vi "Open_Refs.vi"(10 "Refs_Destination_Cabine":refnum<vi>[](array[refnum]), 11 "Ref_Appel_Couloir":refnum<vi>[](array[refnum])) -> (3 "Donnees_Globale_Out":T1)   [LabVIEW 2019]
uses:
  Asc_State_Inputs.ctl
  Etat_Asc.ctl
  <vilib>/FPGAPlugInAG/myRIO-1900/niLvFpga_Open_myRIO-1900.vi
  <vilib>/rvi/interface/common/dynamic/niFpgaDynamicAddResources.vi
  <vilib>/Utility/error.llb/Error Cluster From Error Code.vi
  <vilib>/rvi/errors/niLvFpgaAdjustHostInterfaceError.vi
  <vilib>/rvi/interface/nirviOpenFPGA/nirviOpenFPGA.xnode
  FPGA Bitfiles/ascenceur_FPGATarget_FPGAMain_7v9Jr2n8zuw.lvbitx
  L298N/FPGA_Main.vi
  <vilib>/rvi/interface/nirviReadWriteControl/nirviReadWriteControl.xnode
  <vilib>/myRIO/Common/Instrument Driver Framework/myRIO v1.0/DIO/typedefs/DIO Channels Enum.ctl
  <vilib>/myRIO/Common/Instrument Driver Framework/myRIO v1.0/DIO/typedefs/DIO Channels List.ctl
  <vilib>/myRIO/Common/Instrument Driver Framework/Utilities/typedefs/Generic FPGA Reference.ctl
  <vilib>/myRIO/Common/Instrument Driver Framework/Utilities/typedefs/myRIO v1.0 Reference.ctl
  <vilib>/myRIO/Common/Instrument Driver Framework/Utilities/typedefs/Hardware Version Enum.ctl
  <vilib>/myRIO/Common/Instrument Driver Framework/Utilities/typedefs/myRIO Generic Hardware Reference.ctl
  <vilib>/myRIO/Instrument Drivers/Onboard IO/DIO/typedefs/DIO Reference.ctl
  <vilib>/myRIO/Instrument Drivers/Onboard IO/DIO/DIO.lvlib
  <vilib>/userDefined/High Color/nirio_resource_hc.ctl
  <vilib>/myRIO/Common/Instrument Driver Framework/myRIO v1.0/DIO/vis/myRIO v1.1 Open DIO.vi
  <vilib>/myRIO/Instrument Drivers/Onboard IO/DIO/vis/myRIO DIO Open.xnode
  L298N_Driver/L298N_Ref_Type.ctl
  NiFpgaLv.dll
  <vilib>/rvi/interface/Simulation/niFpgaSimulationCallBeginRW.vi
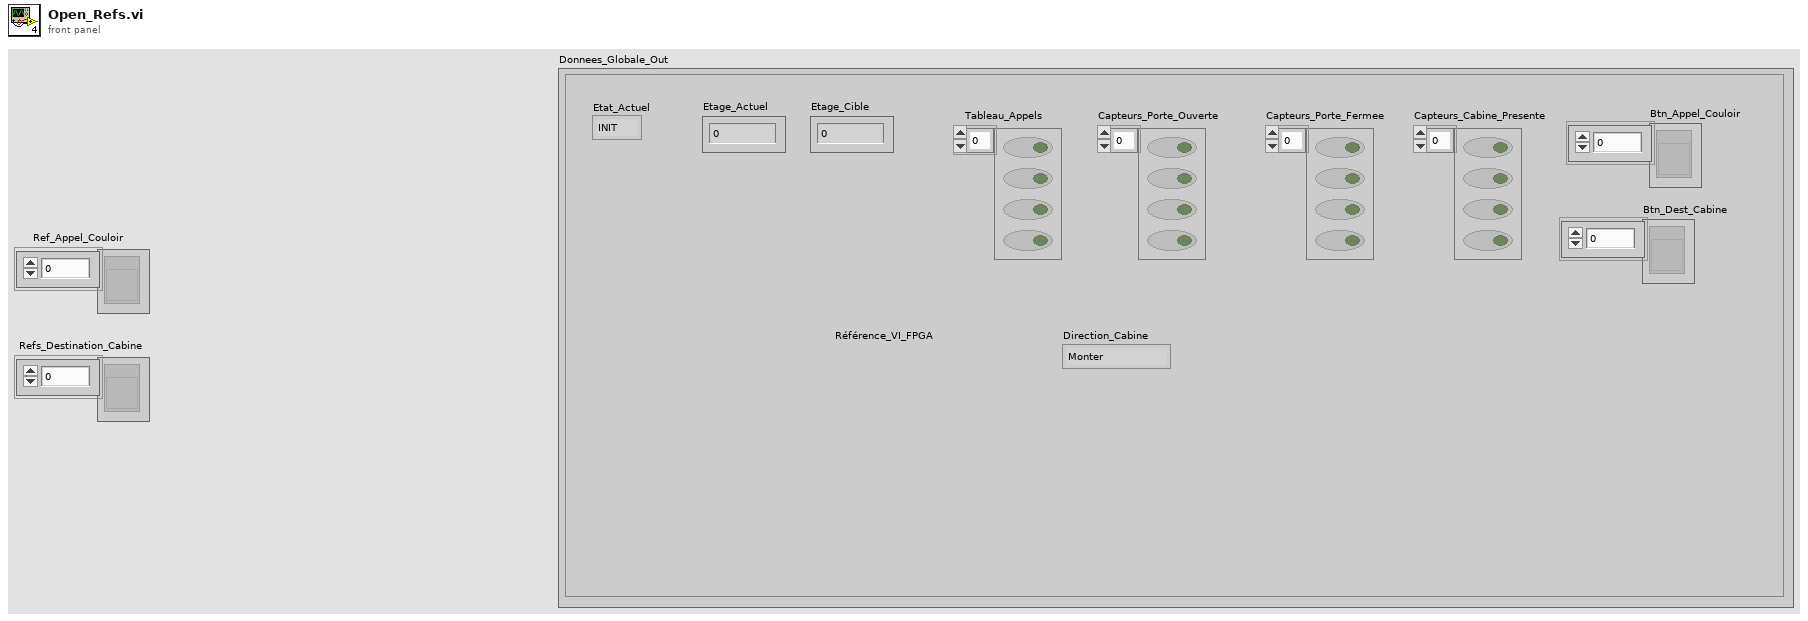
[diagram p1: front panel]
types:
  T1 = typedef "Asc_State_Inputs.ctl" = cluster{"Etage_Actuel":i32, "Etat_Actuel":T2, "Etage_Cible":i32, "Tableau_Appels":bool[], "Capteurs_Porte_Ouverte":bool[], "Capteurs_Porte_Fermee":bool[], "Capteurs_Cabine_Presente":bool[], "Btn_Appel_Couloir":refnum<vi>[], "Btn_Dest_Cabine":refnum<vi>[], "Référence_VI_FPGA":refnum<k20>, "Direction_Cabine":enum16{"Monter", "Descendre", "Arreter"}}
  T2 = typedef "Etat_Asc.ctl" = enum16{"INIT", "REPOS", "DEPLACEMENT", "OUVERTURE_PORTE", "ATTENTE_TEMPO", "FERMETURE_PORTE", "ARRET_URGENCE"}
  T3 = typedef "L298N_Ref_Type.ctl" = cluster{"DIO_Ref_Montee":T4, "DIO_Ref_Descente":T4}
  T4 = typedef "DIO.lvlib/DIO Reference.ctl" = cluster{"myRIO Reference":T5, "DIO Channels List":T9}
  T5 = typedef "myRIO Generic Hardware Reference.ctl" = cluster{"myRIO Model":T6, "myRIO Hardware Reference":T7}
  T6 = typedef "Hardware Version Enum.ctl" = enum16{"Unknown", "myRIO-1900", "myRIO-1950", "roboRIO", "NI ELVIS RIO CM", "ELVIS III"}
  T7 = typedef "myRIO v1.0 Reference.ctl" = cluster{"Generic FPGA Reference":T8, "Allow multiple opens":bool}
  T8 = typedef "Generic FPGA Reference.ctl" = refnum<k20>
  T9 = typedef "DIO Channels List.ctl" = T10[]
  T10 = typedef "DIO Channels Enum.ctl" = enum16{"Not Connected", "C/DIO0", "C/DIO1", "C/DIO2", "C/DIO3", "C/DIO4", "C/DIO5", "C/DIO6", "C/DIO7", "A/DIO0", "A/DIO1", "A/DIO2", "A/DIO3", "A/DIO4", "A/DIO5", "A/DIO6", "A/DIO7", "A/DIO8", "A/DIO9", "A/DIO10", "A/DIO11", "A/DIO12", "A/DIO13", "A/DIO14", "A/DIO15", "A/DIO16", "A/DIO17", "A/DIO18", "A/DIO19", "B/DIO0", "B/DIO1", "B/DIO2", "B/DIO3", "B/DIO4", "B/DIO5", "B/DIO6", "B/DIO7", "B/DIO8", "B/DIO9", "B/DIO10", "B/DIO11", "B/DIO12", "B/DIO13", "B/DIO14", "B/DIO15", "B/DIO16", "B/DIO17", "B/DIO18", "B/DIO19", "LED0", "LED1", "LED2", "LED3", "Button0", "DIO/DIO0", "DIO/DIO1", "DIO/DIO2", "DIO/DIO3", "DIO/DIO4", "DIO/DIO5", "DIO/DIO6", "DIO/DIO7", "DIO/DIO8", "DIO/DIO9", "SPI/CS0", "SPI/CS1", "SPI/CS2", "SPI/CS3", "LED RADIO (Green)", "LED RADIO (Red)", "LED COMM (Green)", "LED COMM (Red)", "LED MODE (Green)", "LED MODE (Red)"}
  T11 = typedef "nirio_resource_hc.ctl" = tag
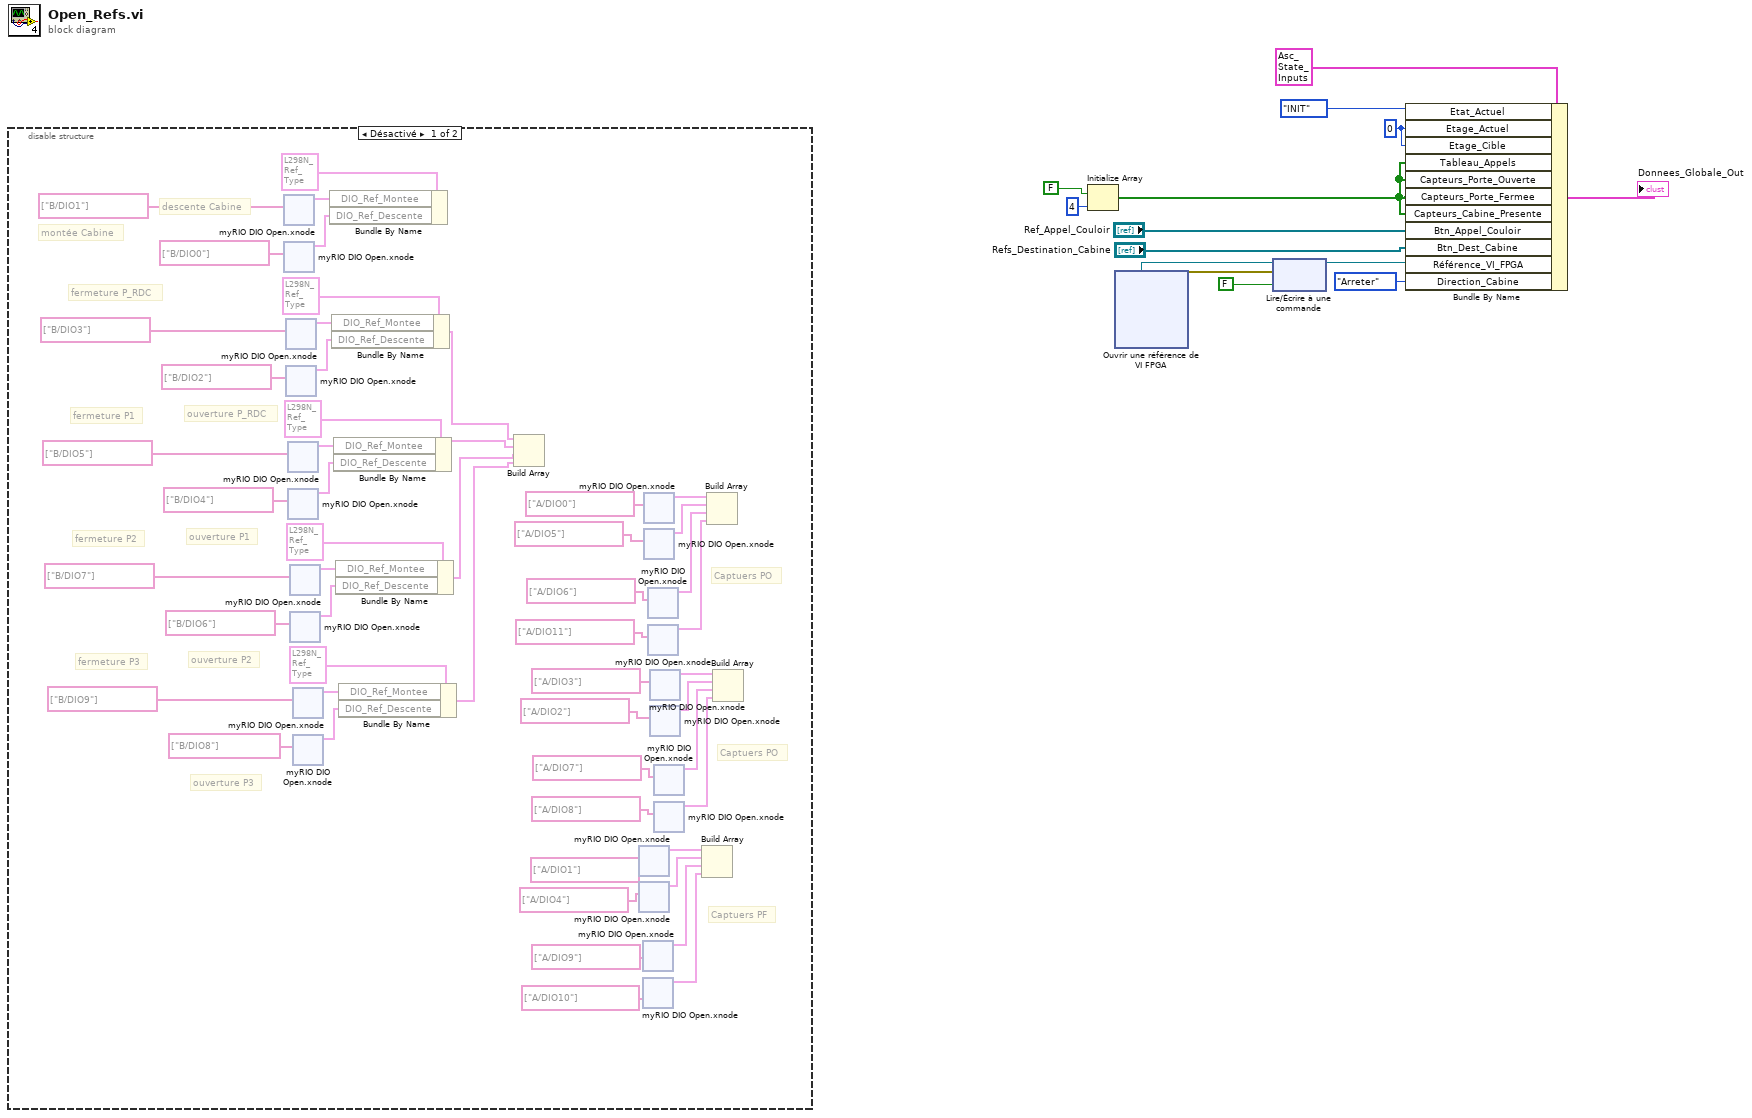
[diagram p0: block diagram]
diagram:
  w7 = 0 ("Etage_Actuel")
  n1 = disable-structure shown="Désactivé" {
    frame Disabled {
      # "montée Cabine"
      # "descente Cabine"
      # "Captuers PO"
      # "Captuers PO"
      # "Captuers PF"
      # "fermeture P3"
      # "ouverture P3"
      # "fermeture P2"
      # "ouverture P2"
      # "fermeture P1"
      # "ouverture P1"
      # "fermeture P_RDC"
      # "ouverture P_RDC"
      n2 = xnode "myRIO DIO Open.xnode"("Channel Names"=tag[] ["B/DIO1"]) -> ("DIO Ref Out"=w17:T4)  [unwired: 2 in, 1 out]
      n3 = xnode "myRIO DIO Open.xnode"("Channel Names"=tag[] ["B/DIO0"]) -> ("DIO Ref Out"=w16:T4)  [unwired: 2 in, 1 out]
      n4 = xnode "myRIO DIO Open.xnode"("Channel Names"=tag[] ["B/DIO3"]) -> ("DIO Ref Out"=w65:T4)  [unwired: 2 in, 1 out]
      n5 = xnode "myRIO DIO Open.xnode"("Channel Names"=tag[] ["B/DIO2"]) -> ("DIO Ref Out"=w66:T4)  [unwired: 2 in, 1 out]
      n6 = xnode "myRIO DIO Open.xnode"("Channel Names"=tag[] ["B/DIO5"]) -> ("DIO Ref Out"=w60:T4)  [unwired: 2 in, 1 out]
      n7 = xnode "myRIO DIO Open.xnode"("Channel Names"=tag[] ["B/DIO4"]) -> ("DIO Ref Out"=w59:T4)  [unwired: 2 in, 1 out]
      n8 = xnode "myRIO DIO Open.xnode"("Channel Names"=tag[] ["B/DIO7"]) -> ("DIO Ref Out"=w55:T4)  [unwired: 2 in, 1 out]
      n9 = xnode "myRIO DIO Open.xnode"("Channel Names"=tag[] ["B/DIO6"]) -> ("DIO Ref Out"=w56:T4)  [unwired: 2 in, 1 out]
      n10 = xnode "myRIO DIO Open.xnode"("Channel Names"=tag[] ["B/DIO9"]) -> ("DIO Ref Out"=w50:T4)  [unwired: 2 in, 1 out]
      n11 = xnode "myRIO DIO Open.xnode"("Channel Names"=tag[] ["B/DIO8"]) -> ("DIO Ref Out"=w49:T4)  [unwired: 2 in, 1 out]
      n12 = Bundle By Name(cluster=T3 {"DIO_Ref_Montee"={"myRIO Reference"={"myRIO Model"=enum."Unknown", "myRIO Hardware Reference"={"Generic FPGA Reference"=refnum, "Allow multiple opens"=FALSE}}, "DIO Channels List"=[]}, "DIO_Ref_Descente"={"myRIO Reference"={"myRIO Model"=enum."Unknown", "myRIO Hardware Reference"={"Generic FPGA Reference"=refnum, "Allow multiple opens"=FALSE}}, "DIO Channels List"=[]}} ("Cluster 2"), "DIO_Ref_Montee"=w17, "DIO_Ref_Descente"=w16) -> ()  [unwired: 1 out]
      n13 = Bundle By Name(cluster=T3 {"DIO_Ref_Montee"={"myRIO Reference"={"myRIO Model"=enum."Unknown", "myRIO Hardware Reference"={"Generic FPGA Reference"=refnum, "Allow multiple opens"=FALSE}}, "DIO Channels List"=[]}, "DIO_Ref_Descente"={"myRIO Reference"={"myRIO Model"=enum."Unknown", "myRIO Hardware Reference"={"Generic FPGA Reference"=refnum, "Allow multiple opens"=FALSE}}, "DIO Channels List"=[]}} ("Cluster 2"), "DIO_Ref_Montee"=w65, "DIO_Ref_Descente"=w66) -> (w47:T3)
      n14 = Bundle By Name(cluster=T3 {"DIO_Ref_Montee"={"myRIO Reference"={"myRIO Model"=enum."Unknown", "myRIO Hardware Reference"={"Generic FPGA Reference"=refnum, "Allow multiple opens"=FALSE}}, "DIO Channels List"=[]}, "DIO_Ref_Descente"={"myRIO Reference"={"myRIO Model"=enum."Unknown", "myRIO Hardware Reference"={"Generic FPGA Reference"=refnum, "Allow multiple opens"=FALSE}}, "DIO Channels List"=[]}} ("Cluster 2"), "DIO_Ref_Montee"=w60, "DIO_Ref_Descente"=w59) -> (w46:T3)
      n15 = Bundle By Name(cluster=T3 {"DIO_Ref_Montee"={"myRIO Reference"={"myRIO Model"=enum."Unknown", "myRIO Hardware Reference"={"Generic FPGA Reference"=refnum, "Allow multiple opens"=FALSE}}, "DIO Channels List"=[]}, "DIO_Ref_Descente"={"myRIO Reference"={"myRIO Model"=enum."Unknown", "myRIO Hardware Reference"={"Generic FPGA Reference"=refnum, "Allow multiple opens"=FALSE}}, "DIO Channels List"=[]}} ("Cluster 2"), "DIO_Ref_Montee"=w55, "DIO_Ref_Descente"=w56) -> (w45:T3)
      n16 = Bundle By Name(cluster=T3 {"DIO_Ref_Montee"={"myRIO Reference"={"myRIO Model"=enum."Unknown", "myRIO Hardware Reference"={"Generic FPGA Reference"=refnum, "Allow multiple opens"=FALSE}}, "DIO Channels List"=[]}, "DIO_Ref_Descente"={"myRIO Reference"={"myRIO Model"=enum."Unknown", "myRIO Hardware Reference"={"Generic FPGA Reference"=refnum, "Allow multiple opens"=FALSE}}, "DIO Channels List"=[]}} ("Cluster 2"), "DIO_Ref_Montee"=w50, "DIO_Ref_Descente"=w49) -> (w44:T3)
      n17 = Build Array(w47, w46, w45, w44) -> ()  [unwired: 1 out]
      n18 = xnode "myRIO DIO Open.xnode"("Channel Names"=tag[] ["A/DIO1"]) -> ("DIO Ref Out"=w28:T4)  [unwired: 2 in, 1 out]
      n19 = xnode "myRIO DIO Open.xnode"("Channel Names"=tag[] ["A/DIO4"]) -> ("DIO Ref Out"=w31:T4)  [unwired: 2 in, 1 out]
      n20 = xnode "myRIO DIO Open.xnode"("Channel Names"=tag[] ["A/DIO9"]) -> ("DIO Ref Out"=w30:T4)  [unwired: 2 in, 1 out]
      n21 = xnode "myRIO DIO Open.xnode"("Channel Names"=tag[] ["A/DIO10"]) -> ("DIO Ref Out"=w29:T4)  [unwired: 2 in, 1 out]
      n22 = xnode "myRIO DIO Open.xnode"("Channel Names"=tag[] ["A/DIO0"]) -> ("DIO Ref Out"=w27:T4)  [unwired: 2 in, 1 out]
      n23 = xnode "myRIO DIO Open.xnode"("Channel Names"=tag[] ["A/DIO5"]) -> ("DIO Ref Out"=w24:T4)  [unwired: 2 in, 1 out]
      n24 = xnode "myRIO DIO Open.xnode"("Channel Names"=tag[] ["A/DIO6"]) -> ("DIO Ref Out"=w25:T4)  [unwired: 2 in, 1 out]
      n25 = xnode "myRIO DIO Open.xnode"("Channel Names"=tag[] ["A/DIO11"]) -> ("DIO Ref Out"=w26:T4)  [unwired: 2 in, 1 out]
      n26 = xnode "myRIO DIO Open.xnode"("Channel Names"=tag[] ["A/DIO3"]) -> ("DIO Ref Out"=w43:T4)  [unwired: 2 in, 1 out]
      n27 = xnode "myRIO DIO Open.xnode"("Channel Names"=tag[] ["A/DIO2"]) -> ("DIO Ref Out"=w40:T4)  [unwired: 2 in, 1 out]
      n28 = xnode "myRIO DIO Open.xnode"("Channel Names"=tag[] ["A/DIO7"]) -> ("DIO Ref Out"=w41:T4)  [unwired: 2 in, 1 out]
      n29 = xnode "myRIO DIO Open.xnode"("Channel Names"=tag[] ["A/DIO8"]) -> ("DIO Ref Out"=w42:T4)  [unwired: 2 in, 1 out]
      n30 = Build Array(w28, w31, w30, w29) -> ()  [unwired: 1 out]
      n31 = Build Array(w27, w24, w25, w26) -> ()  [unwired: 1 out]
      n32 = Build Array(w43, w40, w41, w42) -> ()  [unwired: 1 out]
    }
    frame Enabled {
    }
  }
  n33 = Initialize Array(FALSE, 4 ("taille de la dimension")) -> (w9:bool[])
  n34 = xnode "Ouvrir une référence de VI FPGA"() -> ("Référence de VI FPGA en sortie"=w5:refnum<k20>, "sortie d'erreur"=w4:errorcluster)  [unwired: 2 in]
  n35 = xnode "Lire/Écrire à une commande"("Référence de VI FPGA en entrée"=w5, "entrée d'erreur"=w4, "STOP"=FALSE) -> ("Référence de VI FPGA en sortie"=w2:refnum<k20>)  [unwired: 1 out]
  n36 = Bundle By Name(cluster=T1 {"Etage_Actuel"=0, "Etat_Actuel"=enum."INIT", "Etage_Cible"=0, "Tableau_Appels"=[], "Capteurs_Porte_Ouverte"=[], "Capteurs_Porte_Fermee"=[], "Capteurs_Cabine_Presente"=[], "Btn_Appel_Couloir"=[], "Btn_Dest_Cabine"=[], "Référence_VI_FPGA"=refnum, "Direction_Cabine"=enum."Monter"} ("State_Params"), "Etat_Actuel"=Etat_Asc."INIT", "Etage_Actuel"=w7, "Etage_Cible"=w7, "Tableau_Appels"=w9, "Capteurs_Porte_Ouverte"=w9, "Capteurs_Porte_Fermee"=w9, "Capteurs_Cabine_Presente"=w9, "Btn_Appel_Couloir"="Ref_Appel_Couloir", "Btn_Dest_Cabine"="Refs_Destination_Cabine", "Référence_VI_FPGA"=w2, "Direction_Cabine"=enum16{"Monter", "Descendre", "Arreter"}."Arreter") -> (→"Donnees_Globale_Out":T1)
